vi "startup.vi"(8 "error in (no error)":errorcluster, 10 "Listbox in":refnum<vi>, 11 "ExperimentRunner in":refnum<class "ExperimentRunner.lvclass">) -> (0 "error out":errorcluster, 2 "Listbox out":refnum<vi>, 3 "ExperimentRunner out":refnum<class "ExperimentRunner.lvclass">)   [LabVIEW 2009, in "Views.lvlib" / "ExperimentControl.lvlib" / "ExperimentRunner.lvclass"]
uses:
  ExperimentRunner.lvclass
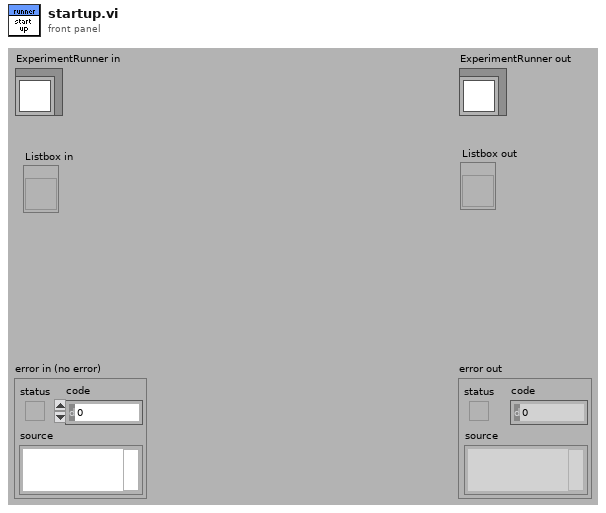
[diagram p1: front panel]
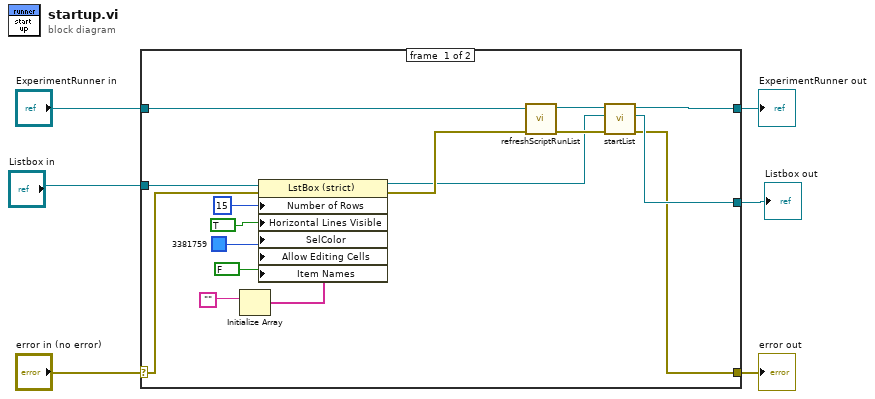
[diagram p0: block diagram]
diagram:
  n1 = case shown="No Error" "error in (no error)" {
    selector: "error in (no error)" -> [w19 w24]
    tunnel: [w7 w24] -> w5
    tunnel: [w10 w23] -> w3
    tunnel: "ExperimentRunner in" -> [w16 w23]
    tunnel: "Listbox in" -> [w18 _]
    tunnel: [w9 _] -> w2
    frame #0 {
      n2 = Initialize Array("") -> (w13:string[])  [unwired: 1 in]
      n3 = property on="Property Node" class="LstBox (strict)"(reference=w18, error in=w19, "Number of Rows"=15, "Horizontal Lines Visible"=TRUE, "SelColor"=u32 3381759, "Allow Editing Cells"=FALSE, "Item Names"=w13) -> (reference out=w8:refnum<vi>, error out=w15:errorcluster)
      n4 = call "refreshScriptRunList.vi"("error in (no error)"=w15, "ExperimentRunner in"=w16) -> ("error out"=w12:errorcluster, "ExperimentRunner out"=w11:refnum<class "ExperimentRunner.lvclass">)  [unwired: 8 in]
      n5 = call "startList.vi"("error in (no error)"=w12, "Listbox"=w8, "ExperimentRunner in"=w11) -> ("error out"=w7:errorcluster, "Listbox out"=w9:refnum<vi>, "ExperimentRunner out"=w10:refnum<class "ExperimentRunner.lvclass">)  [unwired: 6 in]
    }
    frame #1 {
    }
  }
  "error out" <- w5
  "ExperimentRunner out" <- w3
  "Listbox out" <- w2
